vi "GetTaskFormList.vi"(11 "Listbox":refnum<vi>) -> (1 "Label":string[](array[string]), 2 "Time":string[](array[string]), 3 "Tasks":string[](array[string]))   [LabVIEW 2025, in "DAQ_Module.lvlib" / "DAQ_Module.lvclass"]
uses:
  DAQ_Module.lvclass
  DAQ_Module.lvclass/DAQ_Module.ctl
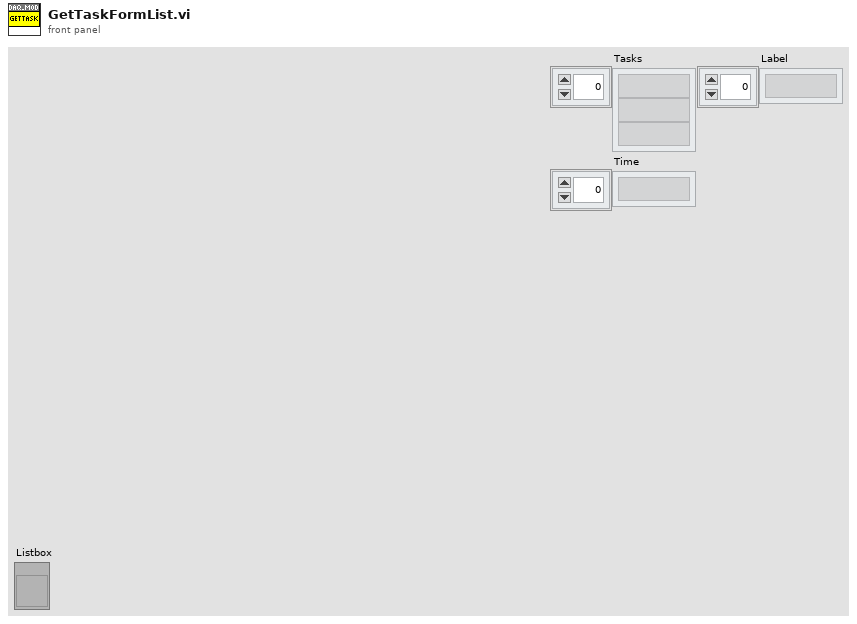
[diagram p1: front panel]
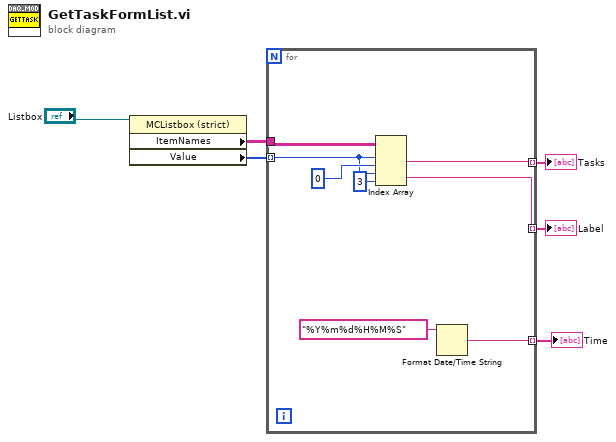
[diagram p0: block diagram]
diagram:
  n1 = property class="MCListbox (strict)"(reference="Listbox") -> ("ItemNames"=w5:string[][], "Value"=w4:i32[])  [unwired: 1 in, 2 out]
  n2 = for {
    tunnel: w5 -> [w14]
    tunnel: w4 -> [w9] mode=indexing
    tunnel: [w12] -> w3 mode=indexing
    tunnel: [w10] -> w2 mode=indexing
    tunnel: [w7] -> w1 mode=indexing
    n3 = Index Array(array=w14, index (row) #1=w9, index (col) #1=0 ("disabled index (col)"), index (row) #2=w9, index (col) #2=3 ("disabled index (col)")) -> (element #1=w12:string, element #2=w7:string)
    n4 = Format Date/Time String(time format string (%c)="%Y%m%d%H%M%S") -> (date/time string=w10:string)  [unwired: 2 in]
  }
  "Tasks" <- w3
  "Time" <- w2
  "Label" <- w1
